vi "BRig_dataMTrig_SolenoidCal_L.vi"() -> (2 "output_SolenoidCal_L":i32)   [LabVIEW 2014]
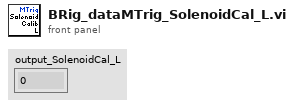
[diagram p1: front panel]
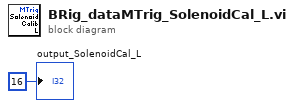
[diagram p0: block diagram]
diagram:
  "output_SolenoidCal_L" <- 16 ("output_iBlock")
